vi "Close_Top_Level_VIs.vi"(8 "error in (no error)":errorcluster, 10 "Top-Level VIs":refnum<vi>[](array[refnum]), 11 "build in":refnum<class "AB_SourceDistribution.lvclass">) -> (0 "error out":errorcluster, 3 "build out":refnum<class "AB_SourceDistribution.lvclass">)   [LabVIEW 2020, in "AB_SourceDistribution.lvclass"]
uses:
  <vilib>/AppBuilder/AB_Classes/SourceDistribution/AB_SourceDistribution.lvclass
  e:/builds/penguin/labview/branches/2020/dev/dist/vi.lib/AppBuilder/AB_Classes/Build/AB_Build.lvclass
  <vilib>/AppBuilder/AB_Classes/Build/AB_Build.lvclass
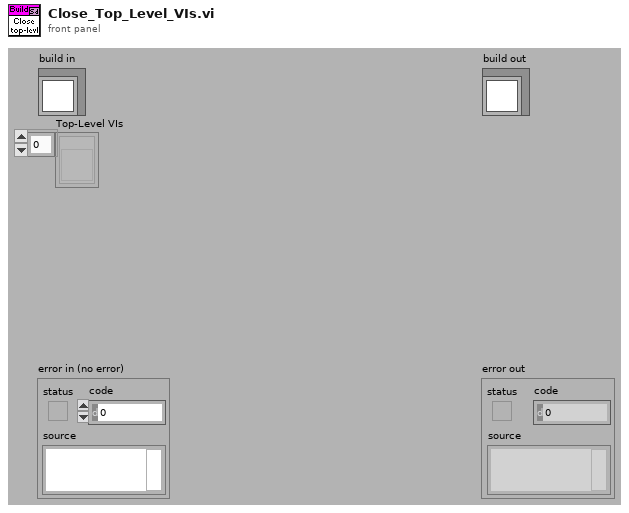
[diagram p1: front panel]
types:
  T1 = typedef "AB_Build.ctl" = cluster{"buildSpecName":string, "buildSpecDescription":string, "destinations":refnum<class "AB_Destination.lvclass">[], "exclusionOption":T2, "defaultLanguage":string, "supportedLanguages":string[], "excludedDirectories":path[], "buildContext":refnum<vi>, "buildObject":T3, "preview":bool, "programatic":bool, "progressBarEvents":T4, "userLog_Path":path, "preActionID":string, "preAction_Path":path, "postActionID":string, "postAction_Path":path, "eng_checkForBrokenVIs?":bool, "eng_verboseLinkerErrors?":bool, "localDest_Path":path, "targetDest_Path":path, "removeVIObject":u16, "cache":refnum<class "PreviewCache.lvclass">, "use cache":bool, "previewCache_ID":string, "buildCache_ID":string, "eng_TempLocalDest_Path":path, "eng_collectDependencies?":bool, "versionInfo":cluster{"buildVersion":cluster{"major":u16, "minor":u16, "patch":u16, "build":u16}, "autoIncrement":bool}, "eng_enableVIChecksums":bool}
  T2 = typedef "AB_Exclusion_Option.ctl" = cluster{"typedefs":bool, "polymorphicVIs":bool, "unusedLibraryItems":bool, "modifyLibraryFile":bool, "edit-timeDependencies":bool, "inlineVIs":bool, "dependent PPLs":bool, "dependent DLLs":bool}
  T3 = typedef "ItemRef.ctl" = u64
  T4 = typedef "provcom_ProgressBar_Events.ctl" = cluster{"newJob":refnum<user-event>, "newItem":refnum<user-event>, "errorMsg":T5, "cancel":refnum<user-event>}
  T5 = typedef "mxLvBuildError.ctl" = refnum<user-event>
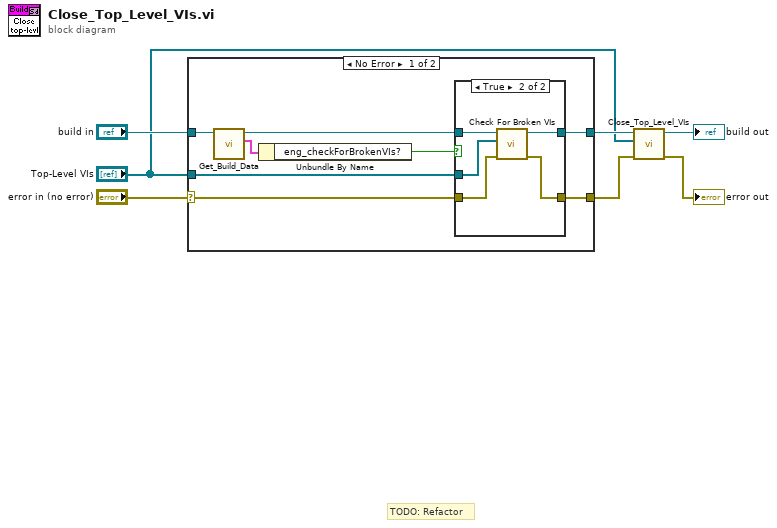
[diagram p0: block diagram]
diagram:
  # "TODO: Refactor"
  n1 = case shown="No Error" "error in (no error)" {
    selector: "error in (no error)" -> [w10 w24]
    tunnel: [w9 w24] -> w3
    tunnel: [w11 w23] -> w2
    tunnel: "build in" -> [w12 w23]
    tunnel: "Top-Level VIs" -> [w8 _]
    frame No Error {
      n2 = call <vilib>:"Get_Build_Data.vi"("Class in"=w12) -> ("data"=w15:T1, "Class out"=w14:refnum<class "AB_SourceDistribution.lvclass">)  [unwired: 8 in, 1 out]
      n3 = Unbundle By Name(w15) -> ("eng_checkForBrokenVIs?"=w13:bool)
      n4 = case shown="True" w13 {
        tunnel: w10 -> [w16 w20]
        tunnel: [w16 w21] -> w9
        tunnel: [w17 w19] -> w11
        tunnel: w14 -> [w17 w22]
        tunnel: w8 -> [_ w18]
        frame False {
        }
        frame True {
          n5 = call <vilib>:"Check For Broken VIs.vi"("error in (no error)"=w20, "Top-Level VIs"=w18, "Class in"=w22) -> ("error out"=w21:errorcluster, "Class out"=w19:refnum<class "AB_SourceDistribution.lvclass">)  [unwired: 7 in]
        }
      }
    }
    frame Error {
    }
  }
  n6 = call-parent "Close_Top_Level_VIs.vi"("error in (no error)"=w3, "Top-Level VIs"="Top-Level VIs", "AB_Build in"=w2) -> ("error out"=→"error out":errorcluster, "AB_Build out"=→"build out":refnum<class "AB_SourceDistribution.lvclass">)  [unwired: 7 in]
